vi "Configure.vi"(0 "Photodiode in":refnum<class "Photodiode.lvclass">, 1 "Timestamp Counter":tag="Dev3/ctr1", 2 "Timestamp Source":tag="/Dev3/10MHzRefClock", 3 "photodiode":tag="Dev3/ai4", 4 "scanimageframesync":tag="Dev3/ai15", 5 "error in (no error)":errorcluster, 6 "Minimum Value":dbl=-10.0 format="%0.2f", 7 "Rate":dbl=10000.0 caption="Sample Rate (Hz)" format="%0.2f", 8 "Maximum Value":dbl=10.0 format="%0.2f", 9 "sample mode":i32(ring)=10123 items=["Finite Samples"=10178, "Continuous Samples"=10123, "Hardware Timed Single Point"=12522], 11 "samples per channel":i32=1000) -> (14 "Photodiode out":refnum<class "Photodiode.lvclass">, 19 "error out":errorcluster)   [LabVIEW 2016, in "Photodiode.lvclass"]
uses:
  Photodiode.lvclass
  Photodiode.lvclass/Photodiode.ctl
  <vilib>/DAQmx/create/channels.llb/DAQmx Create Channel (AI-Voltage-Basic).vi
  <vilib>/DAQmx/configure/timing.llb/DAQmx Timing (Sample Clock).vi
panel:
  in  "data":waveform(dbl)[](array[waveform])
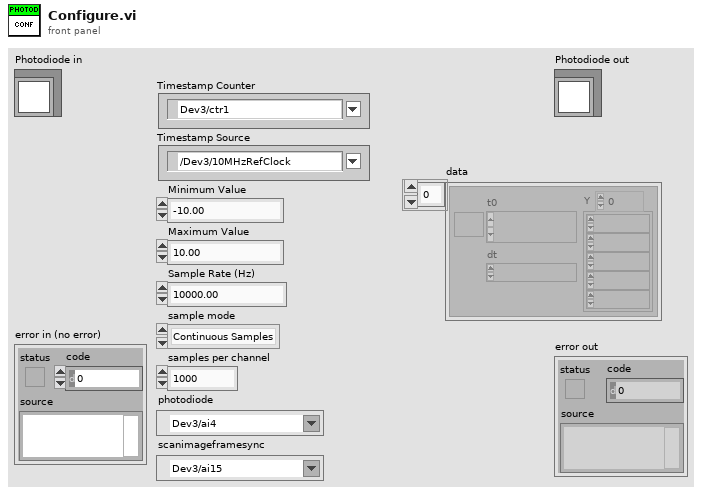
[diagram p1: front panel]
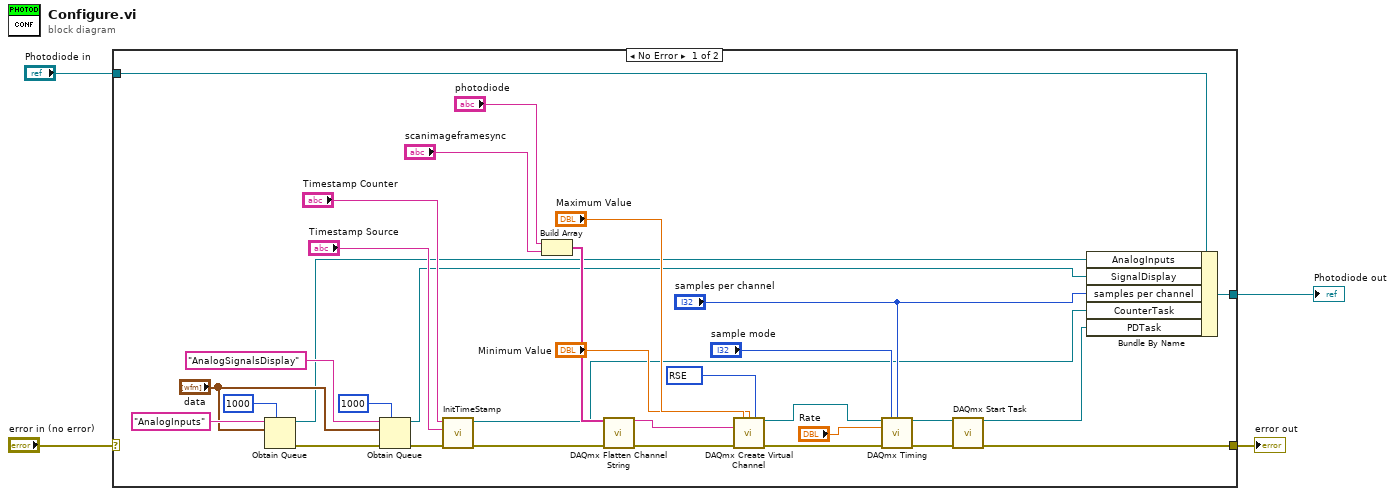
[diagram p0: block diagram]
diagram:
  n1 = case shown="No Error" "error in (no error)" {
    selector: "error in (no error)" -> [_ w38]
    tunnel: [w7 w38] -> w3
    tunnel: [w11 w37] -> w1
    tunnel: "Photodiode in" -> [w12 w37]
    frame No Error {
      w36 = 10083 items=["default"=-1, "RSE"=10083, "NRSE"=10078, "Differential"=10106, "Pseudodifferential"=12529] ("input terminal configuration")
      n2 = Obtain Queue(max queue size (-1, unlimited)=1000, name (unnamed)="AnalogInputs", element data type="data") -> (queue out=w10:refnum<queue>, error out=w23:errorcluster)  [unwired: 2 in, 1 out]
      n3 = Obtain Queue(max queue size (-1, unlimited)=1000, name (unnamed)="AnalogSignalsDisplay", element data type="data", error in (no error)=w23) -> (queue out=w9:refnum<queue>, error out=w15:errorcluster)  [unwired: 1 in, 1 out]
      n4 = call "InitTimeStamp.vi"("error in"=w15, "Input Terminal"="Timestamp Source", "Counter"="Timestamp Counter") -> ("error out"=w14:errorcluster, "task out"=w5:refnum<k21>)  [unwired: 7 in]
      n5 = Build Array("photodiode", "scanimageframesync") -> (w20:tag[])
      n6 = call <vilib>:"DAQmx Flatten Channel String.vi"("names in"=w20, "error in"=w14) -> ("names out"=w19:string, "error out"=w18:errorcluster)  [unwired: 12 in]
      n7 = call-poly <vilib>:"DAQmx Create Virtual Channel.vi"("maximum value"="Maximum Value", "minimum value"="Minimum Value", "input terminal configuration"=w36, "physical channels"=w19, "error in"=w18) -> ("task out"=w34:refnum<k21>, "error out"=w32:errorcluster)  [unwired: 9 in]
      n8 = call-poly <vilib>:"DAQmx Timing.vi"("task/channels in"=w34, "sample mode"="sample mode", "samples per channel"="samples per channel", "rate"="Rate", "error in"=w32) -> ("task out"=w29:refnum<k21>, "error out"=w28:errorcluster)  [unwired: 9 in]
      n9 = call <vilib>:"DAQmx Start Task.vi"("task/channels in"=w29, "error in"=w28) -> ("task out"=w6:refnum<k21>, "error out"=w7:errorcluster)  [unwired: 12 in]
      n10 = Bundle By Name(cluster=w12, "AnalogInputs"=w10, "SignalDisplay"=w9, "samples per channel"="samples per channel", "CounterTask"=w5, "PDTask"=w6) -> (w11:refnum<class "Photodiode.lvclass">)
    }
    frame Error {
    }
  }
  "error out" <- w3
  "Photodiode out" <- w1
